vi "Mult Term By Term Ved3d.vi"(8 "error out":errorcluster, 10 "Vec3d in 2":refnum<class "Vec3d Class.lvclass">, 11 "Vec3d in 1":refnum<class "Vec3d Class.lvclass">) -> (0 "error out 2":errorcluster, 3 "Vec3d Class out":refnum<class "Vec3d Class.lvclass">)   [LabVIEW 2011, in "Vec3d Class.lvclass"]
uses:
  Vec3d Class.lvclass
  Vec3d Class.lvclass/Vec3d Class.ctl
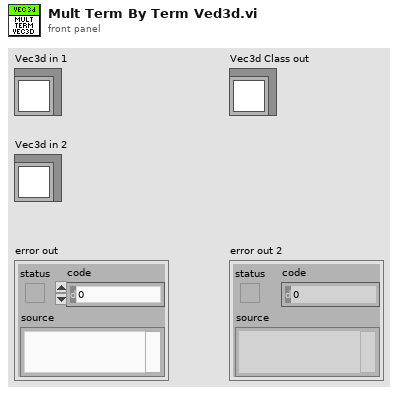
[diagram p1: front panel]
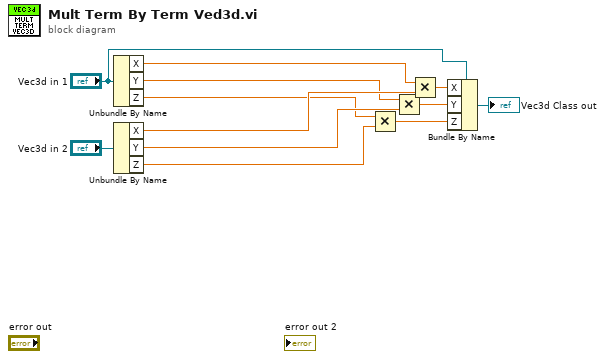
[diagram p0: block diagram]
diagram:
  n1 = Unbundle By Name("Vec3d in 1") -> ("X"=w11:dbl, "Y"=w9:dbl, "Z"=w7:dbl)
  n2 = Unbundle By Name("Vec3d in 2") -> ("X"=w10:dbl, "Y"=w8:dbl, "Z"=w6:dbl)
  n3 = Multiply(x=w7, y=w6) -> (x*y=w2:dbl)
  n4 = Multiply(x=w9, y=w8) -> (x*y=w3:dbl)
  n5 = Multiply(x=w11, y=w10) -> (x*y=w4:dbl)
  n6 = Bundle By Name(cluster="Vec3d in 1", "X"=w4, "Y"=w3, "Z"=w2) -> (→"Vec3d Class out":refnum<class "Vec3d Class.lvclass">)
